vi "8.1.-Momento Invariante de Hu Inicial - Mpq.vi"(1 "q":dbl, 2 "p":dbl, 3 "f(x,y)":dbl[][](array[numeric])) -> (0 "Mpq":dbl)   [LabVIEW 2020]
panel:
  # "Visión Artificial - Momentos Invariantes de Hu\nDiego Cervantes Rodríguez\ndicer0.com"
  # "Momento inicial = Mpq = sum(sum((x^p)*(y^q)*f(x,y)))"
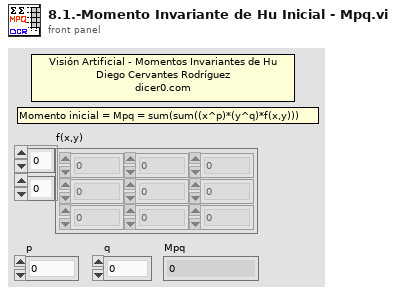
[diagram p1: front panel]
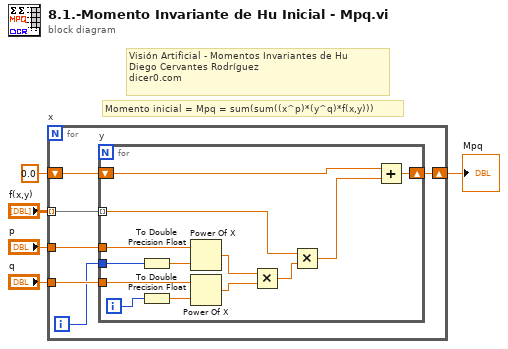
[diagram p0: block diagram]
diagram:
  # "Visión Artificial - Momentos Invariantes de Hu\nDiego Cervantes Rodríguez\ndicer0.com"
  # "Momento inicial = Mpq = sum(sum((x^p)*(y^q)*f(x,y)))"
  n1 = for "x" {
    tunnel: "f(x,y)" -> [w11] mode=indexing
    tunnel: "p" -> [w10]
    tunnel: "q" -> [w9]
    shift-right: [w8] -> w2
    shift-left: 0.0 -> [w7]
    i -> [w6]
    n2 = for "y" {
      tunnel: w11 -> [w14] mode=indexing
      tunnel: w10 -> [w24]
      tunnel: w9 -> [w23]
      shift-right: [w22] -> w8
      shift-left: w7 -> [w13]
      tunnel: w6 -> [w18]
      i -> [w20]
      n3 = To Double Precision Float(number=w18) -> (double precision float=w19:dbl)
      n4 = To Double Precision Float(number=w20) -> (double precision float=w21:dbl)
      n5 = Power Of X(1:w19, 2:w24) -> (0:w16:dbl)
      n6 = Power Of X(1:w21, 2:w23) -> (0:w17:dbl)
      n7 = Multiply(x=w16, y=w17) -> (x*y=w15:dbl)
      n8 = Multiply(x=w14, y=w15) -> (x*y=w12:dbl)
      n9 = Add(x=w13, y=w12) -> (x+y=w22:dbl)
    }
  }
  "Mpq" <- w2
